vi "Convert Rectangle Data to Segment Array.vi"(8 "Error In":errorcluster, 9 "Box Profile Type":T1, 11 "(Rotated) Rectangle Data":i32[](array[numeric])) -> (0 "Error Out":errorcluster, 1 "Median End Points":cluster{"X":dbl, "Y":dbl}[](array[cluster]), 2 "Rectangle End Points":cluster{"X":dbl, "Y":dbl}[](array[cluster]), 3 "Rectange Profile Segments":cluster{"Segment ROI Points":i32[]}[](array[cluster]), 5 "Number of Points":i32)   [LabVIEW 2021, in "Image.lvlib"]
doc: "Converts the array of Rectangle (or Rotated Rectangle) data to an array of structures, each containing an array of (x,y) point coordinates for the corresponding \"cross-section\" segments."
uses:
  Image.lvlib
  Box Profile Type.ctl
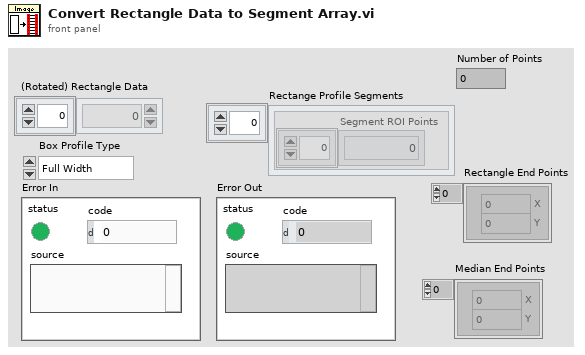
[diagram p1: front panel]
types:
  T1 = typedef "Image.lvlib/Box Profile Type.ctl" = enum16{"Full Width", "Half Width"}
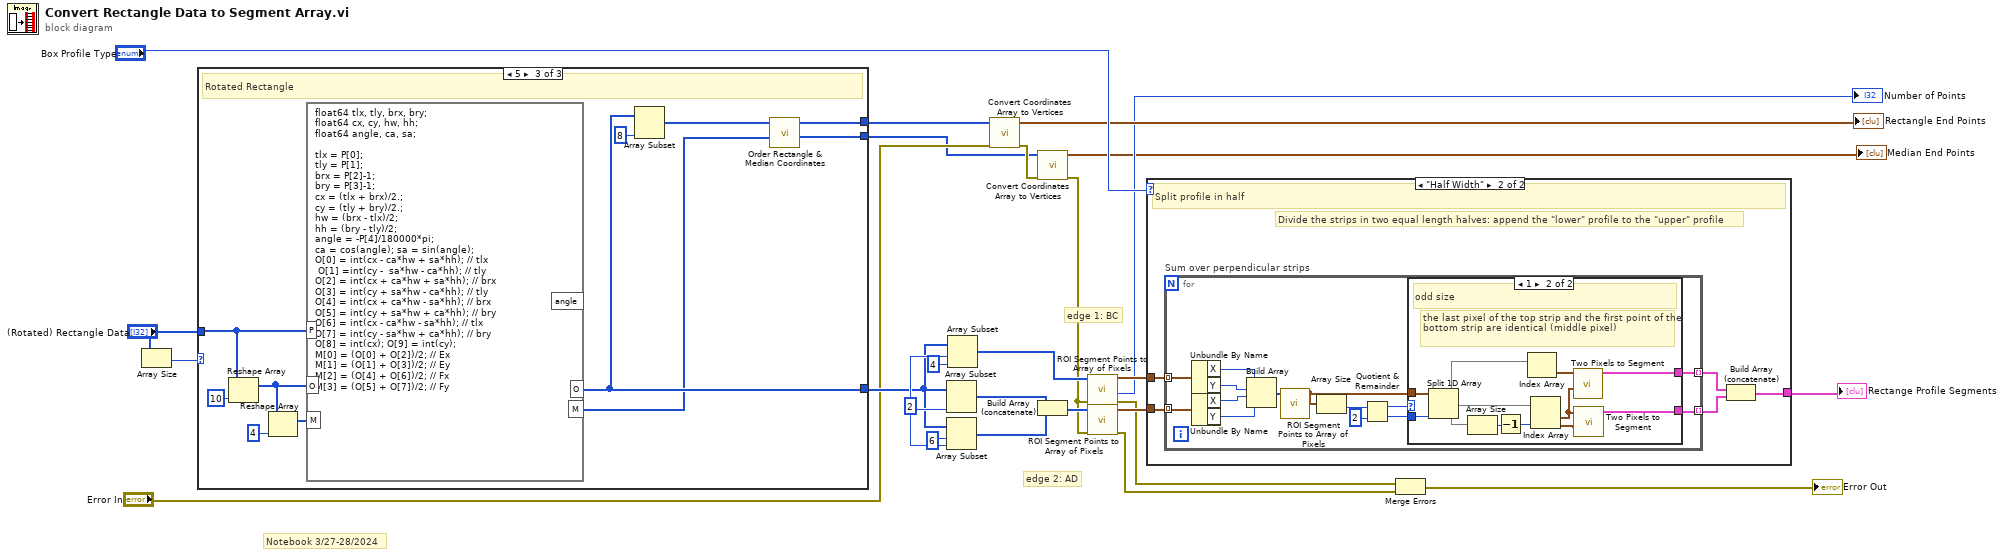
[diagram p0: block diagram]
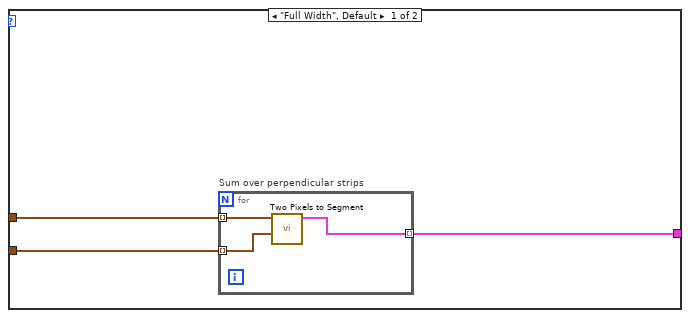
[diagram p2: hidden frame]
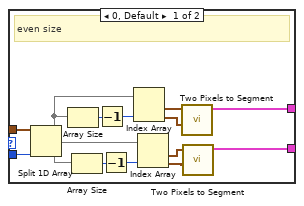
[diagram p3: hidden frame]
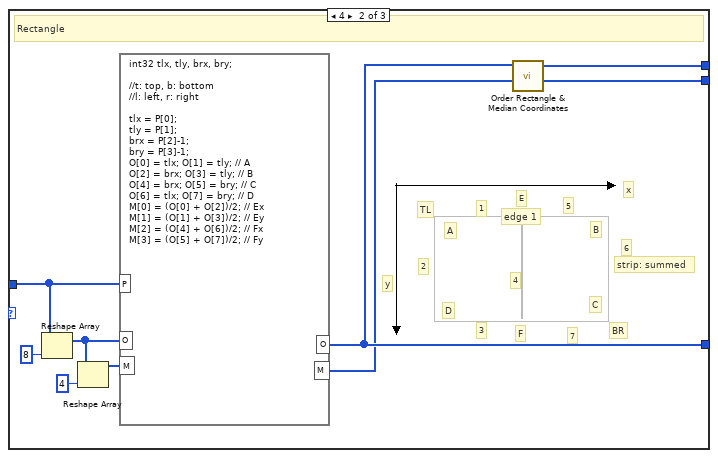
[diagram p5: hidden frame]
diagram:
  w19 = 2 ("length")
  # "edge 2: AD"
  # "edge 1: BC"
  # "Notebook 3/27-28/2024"
  n1 = Array Size(array="(Rotated) Rectangle Data") -> (size(s)=w24:i32)
  n2 = case shown="5" w24 {
    tunnel: "(Rotated) Rectangle Data" -> [_ w34 w45]
    tunnel: [_ w32 w43] -> w9
    tunnel: [_ w27 w36] -> w8
    tunnel: [_ w26 w35] -> w2
    frame 0, Default {
    }
    frame 4 {
      # "7"
      # "6"
      # "5"
      # "4"
      # "3"
      # "2"
      # "1"
      # "F"
      # "E"
      # "strip: summed"
      # "D"
      # "C"
      # "B"
      # "A"
      # "edge 1"
      # "x"
      # "y"
      # "BR"
      # "TL"
      # "Rectangle"
      n3 = Reshape Array(w34, 8 ("dimension size")) -> (w31:i32[])
      n4 = Reshape Array(w31, 4 ("dimension size")) -> (w29:i32[])
      n5 = formula code="int32 tlx, tly, brx, bry;\n\n//t: top, b: bottom\n//l: left, r: right\n\ntlx = P[0];\ntly = P[1];\nbrx = P[2]-1;\nbry = P[3]-1;\nO[0] = tlx; O[1] = tly; // A\nO[2] = brx; O[3] = tly; // B\nO[4] = brx; O[5] = bry; // C\nO[6] = tlx; O[7] = bry; // D\nM[0] = (O[0] + O[2])/2; // Ex\nM[1] = (O[1] + O[3])/2; // Ey\nM[2] = (O[4] + O[6])/2; // Fx\nM[3] = (O[5] + O[7])/2; // Fy"("P"=w34, "O"=w31, "M"=w29) -> ("O"=w32:i32[], "M"=w28:i32[])
      n6 = call "Order Rectangle & Median Coordinates.vi"("EF"=w28, "ABCD"=w32) -> ("Median"=w26:i32[], "Rectangle"=w27:i32[])  [unwired: 8 in]
    }
    frame 5 {
      # "Rotated Rectangle"
      n7 = Reshape Array(w45, 10 ("dimension size")) -> (w40:i32[])
      n8 = Reshape Array(w40, 4 ("dimension size")) -> (w38:i32[])
      n9 = formula code="float64 tlx, tly, brx, bry;\nfloat64 cx, cy, hw, hh;\nfloat64 angle, ca, sa;\n\ntlx = P[0];\ntly = P[1];\nbrx = P[2]-1;\nbry = P[3]-1;\ncx = (tlx + brx)/2.;\ncy = (tly + bry)/2.;\nhw = (brx - tlx)/2;\nhh = (bry - tly)/2;\nangle = -P[4]/180000*pi;\nca = cos(angle); sa = sin(angle);\nO[0] = int(cx - ca*hw + sa*hh); // tlx\n O[1] =int(cy -  sa*hw - ca*hh); // tly\nO[2] = int(cx + ca*hw + sa*hh); // brx\nO[3] = int(cy + sa*hw - ca*hh); // tly\nO[4] = int(cx + ca*hw - sa*hh); // brx\nO[5] = int(cy + sa*hw + ca*hh); // bry\nO[6] = int(cx - ca*hw - sa*hh); // tlx\nO[7] = int(cy - sa*hw + ca*hh); // bry\nO[8] = int(cx); O[9] = int(cy);\nM[0] = (O[0] + O[2])/2; // Ex\nM[1] = (O[1] + O[3])/2; // Ey\nM[2] = (O[4] + O[6])/2; // Fx\nM[3] = (O[5] + O[7])/2; // Fy"("P"=w45, "O"=w40, "M"=w38) -> ("O"=w43:i32[], "M"=w37:i32[])  [unwired: 1 out]
      n10 = Array Subset(array=w43, length=8) -> (w41:i32[])  [unwired: 1 in]
      n11 = call "Order Rectangle & Median Coordinates.vi"("EF"=w37, "ABCD"=w41) -> ("Median"=w35:i32[], "Rectangle"=w36:i32[])  [unwired: 8 in]
    }
  }
  n12 = Array Subset(array=w9, length=w19) -> (w22:i32[])  [unwired: 1 in]
  n13 = Array Subset(array=w9, index=6, length=w19) -> (w20:i32[])
  n14 = Array Subset(array=w9, index=w19, length=4) -> (w17:i32[])
  n15 = call "Convert Coordinates Array to Vertices.vi"("Error In"="Error In", "Coordinates in"=w8) -> ("Error Out"=w4:errorcluster, "Vertices out"=→"Rectangle End Points":cluster{"X":dbl, "Y":dbl}[])  [unwired: 8 in]
  n16 = call "Convert Coordinates Array to Vertices.vi"("Error In"=w4, "Coordinates in"=w2) -> ("Error Out"=w3:errorcluster, "Vertices out"=→"Median End Points":cluster{"X":dbl, "Y":dbl}[])  [unwired: 8 in]
  n17 = Build Array (concatenate)(w22, w20) -> (w21:i32[])
  n18 = call "ROI Segment Points to Array of Pixels.vi"("error in (no error)"=w3, "Segment ROI Points"=w17) -> ("Error Out"=w13:errorcluster, "Number of Points"=→"Number of Points":i32, "Pixels of the Segment"=w16:cluster{"X":i32, "Y":i32}[])  [unwired: 7 in]
  n19 = call "ROI Segment Points to Array of Pixels.vi"("error in (no error)"=w3, "Segment ROI Points"=w21) -> ("Error Out"=w11:errorcluster, "Pixels of the Segment"=w15:cluster{"X":i32, "Y":i32}[])  [unwired: 7 in, 1 out]
  n20 = case shown="\"Half Width\"" "Box Profile Type" {
    tunnel: w16 -> [w48 w55]
    tunnel: w15 -> [w47 w56]
    tunnel: [w46 w52] -> w14
    frame "Full Width", Default {
      n21 = for "Sum over perpendicular strips" {
        tunnel: w48 -> [w51] mode=indexing
        tunnel: w47 -> [w49] mode=indexing
        tunnel: [w50] -> w46 mode=indexing
        n22 = call "Two Pixels to Segment.vi"("Pixel 2"=w49, "Pixel 1"=w51) -> ("Segment 1-2"=w50:cluster{"Array":i32[]})  [unwired: 8 in, 1 out]
      }
    }
    frame "Half Width" {
      # "Divide the strips in two equal length halves: append the \"lower\" profile to the \"upper\" profile"
      # "Split profile in half"
      n23 = for "Sum over perpendicular strips" {
        tunnel: w55 -> [w70] mode=indexing
        tunnel: w56 -> [w69] mode=indexing
        tunnel: [w58] -> w54 mode=indexing
        tunnel: [w57] -> w53 mode=indexing
        n24 = Unbundle By Name(w70) -> ("X"=w68:i32, "Y"=w66:i32)
        n25 = Unbundle By Name(w69) -> ("X"=w65:i32, "Y"=w67:i32)
        n26 = Build Array(w68, w66, w65, w67) -> (w64:i32[])
        n27 = call "ROI Segment Points to Array of Pixels.vi"("Segment ROI Points"=w64) -> ("Pixels of the Segment"=w59:cluster{"X":i32, "Y":i32}[])  [unwired: 8 in, 2 out]
        n28 = Array Size(array=w59) -> (size(s)=w63:i32)
        n29 = Quotient & Remainder(x=w63, y=2) -> (x-y*floor(x/y)=w61:i32, floor(x/y)=w60:i32)
        n30 = case shown="1" w61 {
          tunnel: w60 -> [w83 w94]
          tunnel: w59 -> [w84 w95]
          tunnel: [w77 w91] -> w58
          tunnel: [w71 w86] -> w57
          frame 0, Default {
            # "even size"
            n31 = Split 1D Array(array=w84, index=w83) -> (first subarray=w82:cluster{"X":i32, "Y":i32}[], second subarray=w74:cluster{"X":i32, "Y":i32}[])
            n32 = Array Size(array=w82) -> (size(s)=w81:i32)
            n33 = Array Size(array=w74) -> (size(s)=w75:i32)
            n34 = Decrement(x=w81) -> (x-1=w80:i32)
            n35 = Decrement(x=w75) -> (x-1=w76:i32)
            n36 = Index Array(array=w82, index #2=w80) -> (element #1=w79:cluster{"X":i32, "Y":i32}, element #2=w78:cluster{"X":i32, "Y":i32})  [unwired: 1 in]
            n37 = Index Array(array=w74, index #2=w76) -> (element #1=w73:cluster{"X":i32, "Y":i32}, element #2=w72:cluster{"X":i32, "Y":i32})  [unwired: 1 in]
            n38 = call "Two Pixels to Segment.vi"("Pixel 2"=w78, "Pixel 1"=w79) -> ("Segment 1-2"=w77:cluster{"Array":i32[]})  [unwired: 8 in, 1 out]
            n39 = call "Two Pixels to Segment.vi"("Pixel 2"=w72, "Pixel 1"=w73) -> ("Segment 1-2"=w71:cluster{"Array":i32[]})  [unwired: 8 in, 1 out]
          }
          frame 1 {
            # "the last pixel of the top strip and the first point of the bottom strip are identical (middle pixel)"
            # "odd size"
            n40 = Split 1D Array(array=w95, index=w94) -> (first subarray=w93:cluster{"X":i32, "Y":i32}[], second subarray=w88:cluster{"X":i32, "Y":i32}[])
            n41 = Array Size(array=w88) -> (size(s)=w89:i32)
            n42 = Decrement(x=w89) -> (x-1=w90:i32)
            n43 = Index Array(array=w93) -> (element=w92:cluster{"X":i32, "Y":i32})  [unwired: 1 in]
            n44 = Index Array(array=w88, index #2=w90) -> (element #1=w85:cluster{"X":i32, "Y":i32}, element #2=w87:cluster{"X":i32, "Y":i32})  [unwired: 1 in]
            n45 = call "Two Pixels to Segment.vi"("Pixel 2"=w85, "Pixel 1"=w92) -> ("Segment 1-2"=w91:cluster{"Array":i32[]})  [unwired: 8 in, 1 out]
            n46 = call "Two Pixels to Segment.vi"("Pixel 2"=w87, "Pixel 1"=w85) -> ("Segment 1-2"=w86:cluster{"Array":i32[]})  [unwired: 8 in, 1 out]
          }
        }
      }
      n47 = Build Array (concatenate)(w54, w53) -> (w52:cluster{"Array":i32[]}[])
    }
  }
  "Rectange Profile Segments" <- w14
  n48 = Merge Errors(w13, w11) -> (→"Error Out":errorcluster)
